vi "Post-Build Action.vi"(5 "Files Generated by Build":path[](array[path]), 6 "Top Level/Always Included VIs":path[](array[path]), 7 "Destination Path":path, 8 "error in (no error)":errorcluster, 9 "Target Name":string, 10 "Build Specification Name":string, 11 "Project Path":path) -> (0 "error out":errorcluster)   [LabVIEW 2016, in "Build VIs.lvlib"]
uses:
  Build VIs.lvlib
  <vilib>/Utility/sysdir.llb/System Directory Type.ctl
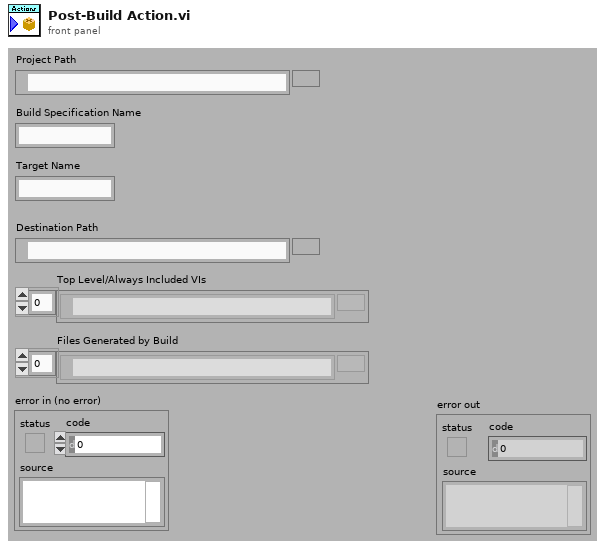
[diagram p1: front panel]
types:
  T1 = typedef "System Directory Type.ctl" = i32
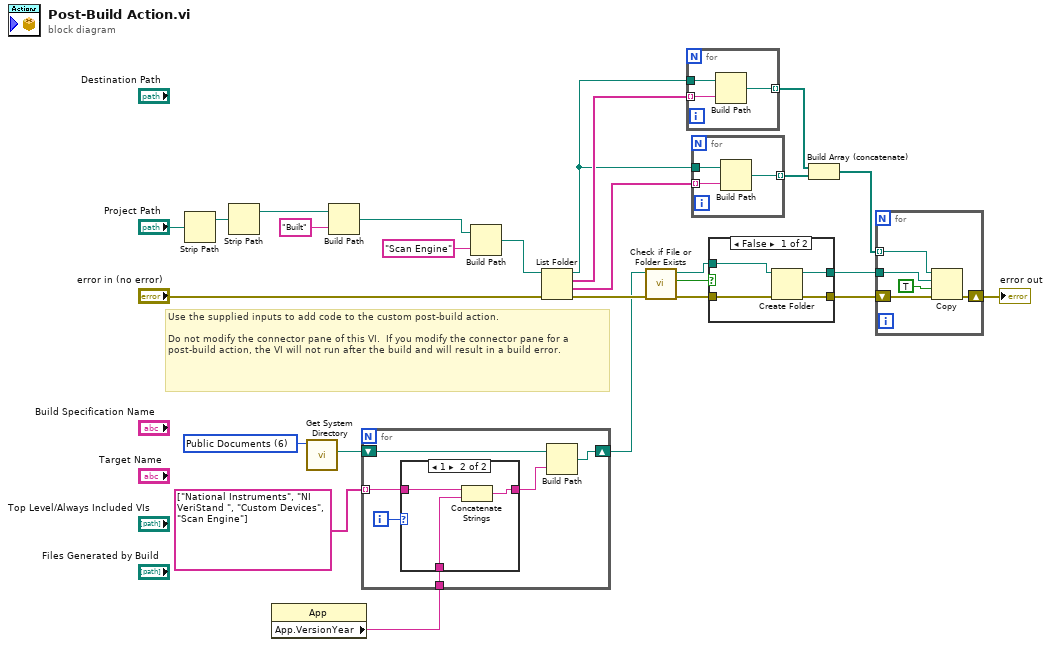
[diagram p0: block diagram]
diagram:
  w7 = T1 6 items=["User Home"=0, "User Desktop"=1, "User Documents"=2, "User Application Data"=3, "User Preferences"=4, "User Temporary"=5, "Public Documents"=6, "Public Application Data"=7, "Public Preferences"=8, "Public Cache"=13, "System Core Libraries"=9, "System Installed Libraries"=10, "Application Files"=11, "Boot Volume Root"=12] ("system directory type")
  # "Use the supplied inputs to add code to the custom post-build action.\n\nDo not modify the connector pane of this VI.  If you modify the connector pane for a post-build action, the VI will not run after the build and will result in a build error."
  n1 = Strip Path(path="Project Path") -> (stripped path=w11:path)  [unwired: 1 out]
  n2 = Strip Path(path=w11) -> (stripped path=w22:path)  [unwired: 1 out]
  n3 = property class="App"() -> ("App.VersionYear"=w3:string)  [unwired: 2 in, 2 out]
  n4 = call <vilib>:"Get System Directory.vi"("system directory type"=w7) -> ("system directory"=w6:path)  [unwired: 10 in]
  n5 = Build Path(base path=w22, name or relative path="Built") -> (appended path=w2:path)
  n6 = for {
    shift-right: [w31] -> w4
    shift-left: w6 -> [w32]
    tunnel: string[] ["National Instruments", "NI VeriStand ", "Custom Devices", "Scan Engine"] -> [w28] mode=indexing
    tunnel: w3 -> [w27]
    i -> [w30]
    n7 = case shown="1" w30 {
      tunnel: [w33 w35] -> w29
      tunnel: w28 -> [w33 w36]
      tunnel: w27 -> [_ w34]
      frame Default {
      }
      frame 1 {
        n8 = Concatenate Strings(w36, w34) -> (w35:string)
      }
    }
    n9 = Build Path(base path=w32, name or relative path=w29) -> (appended path=w31:path)
  }
  n10 = Build Path(base path=w2, name or relative path="Scan Engine") -> (appended path=w10:path)
  n11 = List Folder(path=w10, error in="error in (no error)") -> (path out=w13:path, filenames=w26:string[], folder names=w14:string[], error out=w8:errorcluster)  [unwired: 2 in]
  n12 = call <vilib>:"Check if File or Folder Exists.vi"("error in (no error)"=w8, "path"=w4) -> ("error out"=w17:errorcluster, "file or folder exists?"=w19:bool, "dup path"=w18:path)  [unwired: 7 in]
  n13 = for {
    tunnel: w26 -> [w38] mode=indexing
    tunnel: w13 -> [w39]
    tunnel: [w37] -> w25 mode=indexing
    n14 = Build Path(base path=w39, name or relative path=w38) -> (appended path=w37:path)
  }
  n15 = for {
    tunnel: w14 -> [w41] mode=indexing
    tunnel: w13 -> [w42]
    tunnel: [w40] -> w12 mode=indexing
    n16 = Build Path(base path=w42, name or relative path=w41) -> (appended path=w40:path)
  }
  n17 = case shown="False" w19 {
    tunnel: w18 -> [w46 w48]
    tunnel: w17 -> [w45 w47]
    tunnel: [w44 w48] -> w16
    tunnel: [w43 w47] -> w15
    frame False {
      n18 = Create Folder(path (use dialog)=w46, error in=w45) -> (created path=w44:path, error out=w43:errorcluster)  [unwired: 1 in, 1 out]
    }
    frame True {
    }
  }
  n19 = Build Array (concatenate)(w25, w12) -> (w24:path[])
  n20 = for {
    tunnel: w24 -> [w50] mode=indexing
    shift-right: [w51] -> w1
    shift-left: w15 -> [w52]
    tunnel: w16 -> [w49]
    n21 = Copy(8:w52, 9:TRUE ("overwrite (F)"), 10:w49, 11:w50) -> (0:w51:errorcluster)  [unwired: 1 in, 2 out]
  }
  "error out" <- w1
